vi "SpeedAndAngleToVectorSpeed.vi"(10 "BoatSpeed (m/s)":dbl, 11 "RobotHeading (deg)":dbl) -> (3 "BoatVectorVelocity":T1)   [LabVIEW 2012]
doc: "Spring 2014\n\nReturns the velocity of the boat, given the angle and speed of the boat (m/s)."
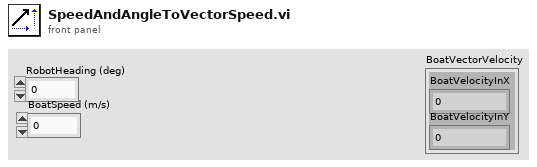
[diagram p1: front panel]
types:
  T1 = cluster{"BoatVelocityInY":dbl, "BoatVelocityInX":dbl}
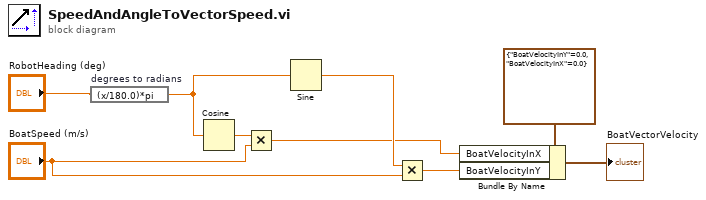
[diagram p0: block diagram]
diagram:
  n1 = expression code="(x/180.0)*pi" "degrees to radians"("RobotHeading (deg)") -> (w1:dbl)
  n2 = Cosine(x=w1) -> (cos(x)=w9:dbl)
  n3 = Multiply(x=w9, y="BoatSpeed (m/s)") -> (x*y=w6:dbl)
  n4 = Sine(x=w1) -> (sin(x)=w8:dbl)
  n5 = Multiply(x=w8, y="BoatSpeed (m/s)") -> (x*y=w5:dbl)
  n6 = Bundle By Name(cluster=T1 {"BoatVelocityInY"=0.0, "BoatVelocityInX"=0.0} ("input cluster"), "BoatVelocityInX"=w6, "BoatVelocityInY"=w5) -> (→"BoatVectorVelocity":T1)
